vi "read.vi"(8 "error in (no error)":errorcluster, 10 "ElectrometerController in":refnum<class "ElectrometerController.lvclass">, 11 "ManualReadingState in":refnum<class "ManualReadingState.lvclass">) -> (0 "error out":errorcluster, 1 "lastMeasure":T1, 2 "ElectrometerController out":refnum<class "ElectrometerController.lvclass">, 3 "ManualReadingState out":refnum<class "ManualReadingState.lvclass">, 4 "newValue":bool)   [LabVIEW 2016, in "ManualReadingState.lvclass"]
uses:
  ManualReadingState.lvclass
  ElectrometerController/ElectrometerController.lvclass
  ts_electrometeruserevents/Typedefs/Reading.ctl
  Electrometer.lvclass
  ts_electrometeruserevents/Typedefs/ElectrometerTypedefs.lvlib
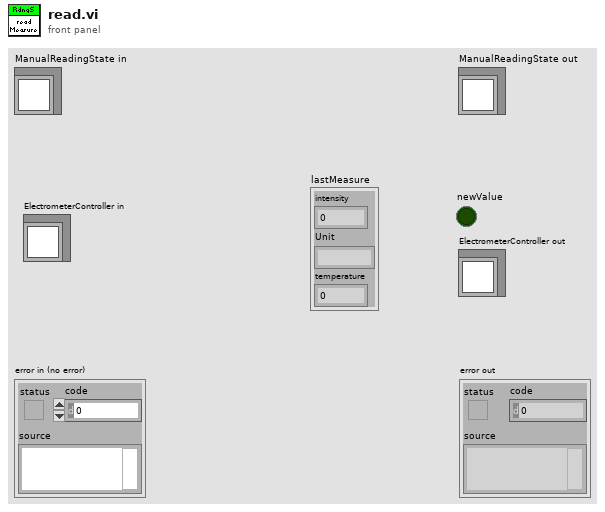
[diagram p1: front panel]
types:
  T1 = typedef "ElectrometerTypedefs.lvlib/Reading.ctl" = cluster{"intensity":dbl, "Unit":string, "temperature":dbl}
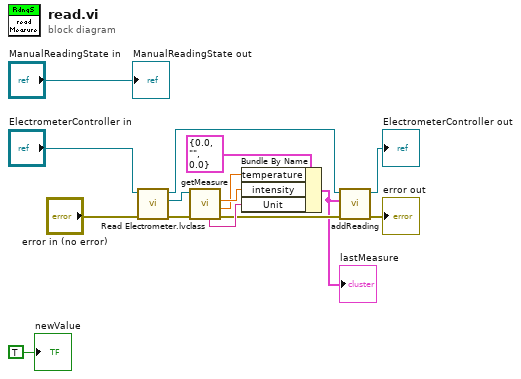
[diagram p0: block diagram]
diagram:
  n1 = call-dynamic "Read Electrometer.lvclass.vi"("error in (no error)"="error in (no error)", "ElectrometerController in"="ElectrometerController in") -> ("error out"=w10:errorcluster, "Electrometer.lvclass"=w11:refnum<class "Electrometer.lvclass">, "ElectrometerController out"=w1:refnum<class "ElectrometerController.lvclass">)  [unwired: 7 in]
  n2 = call "getMeasure.vi"("error in (no error)"=w10, "Electrometer in"=w11) -> ("error out"=w5:errorcluster, "Temperature"=w6:dbl, "Measure"=w8:dbl, "Units"=w9:string)  [unwired: 5 in, 1 out]
  n3 = Bundle By Name(cluster=T1 {"intensity"=0.0, "Unit"="", "temperature"=0.0} ("reading"), "temperature"=w6, "intensity"=w8, "Unit"=w9) -> (w4:T1)
  "lastMeasure" <- w4
  n4 = call "addReading.vi"("error in (no error)"=w5, "reading"=w4, "ElectrometerController in"=w1) -> ("error out"=→"error out":errorcluster, "ElectrometerController out"=→"ElectrometerController out":refnum<class "ElectrometerController.lvclass">)  [unwired: 7 in]
  "ManualReadingState out" <- "ManualReadingState in"
  "newValue" <- TRUE ("newValue")
